vi "Obtain and Save.vi"(8 "error in (no error)":errorcluster, 11 "ErrorLog in":refnum<class "ErrorLog.lvclass">) -> (0 "error out":errorcluster, 3 "ErrorLog out":refnum<class "ErrorLog.lvclass">)   [LabVIEW 2019, in "ErrorLog.lvlib" / "ErrorLog.lvclass"]
uses:
  ErrorLog.lvclass
  LogsAbstract/LogsAbstract.lvclass
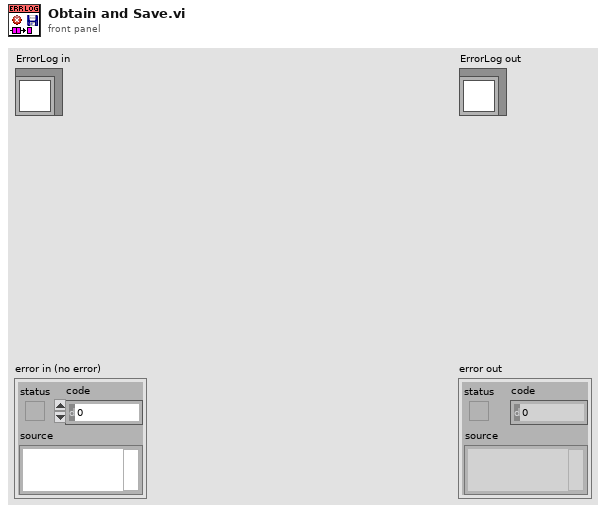
[diagram p1: front panel]
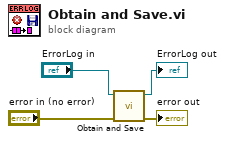
[diagram p0: block diagram]
diagram:
  n1 = call-parent "Obtain and Save.vi"("error in (no error)"="error in (no error)", "LogsAbstract in"="ErrorLog in") -> ("error out"=→"error out":errorcluster, "LogsAbstract out"=→"ErrorLog out":refnum<class "ErrorLog.lvclass">)  [unwired: 8 in]
